vi "PathManager.vi"(11 "path to sequence folder":path) -> (1 "path to Pixmap.bin":path, 2 "path to Pix2Pos.exe":path, 3 "path to Pos.txt":path)   [LabVIEW 2022 SP3]
doc: "This VI builds different useful paths.\n\nIt is used to get the path to pos.txt, Pix2Pos.exe and pixmap.bin.\n\nInput :\n- The path to the sequence's folder\n\nOutputs :\n- The path to Pix2Pos.exe\n- The path to pixmap.bin\n- The path to pos.txt"
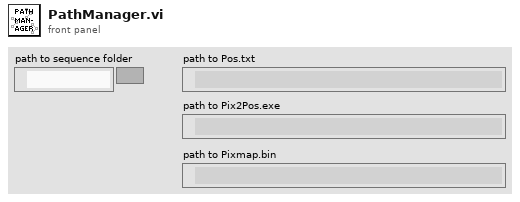
[diagram p1: front panel]
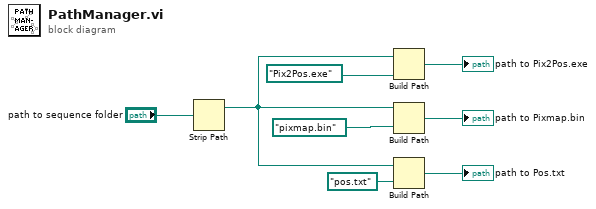
[diagram p0: block diagram]
diagram:
  n1 = Strip Path(path="path to sequence folder") -> (stripped path=w2:path)  [unwired: 1 out]
  n2 = Build Path(base path=w2, name or relative path=path "Pix2Pos.exe") -> (appended path=→"path to Pix2Pos.exe":path)
  n3 = Build Path(base path=w2, name or relative path=path "pixmap.bin") -> (appended path=→"path to Pixmap.bin":path)
  n4 = Build Path(base path=w2, name or relative path=path "pos.txt") -> (appended path=→"path to Pos.txt":path)
